vi "Enable Routing Channel.vi"(8 "error in (no error)":errorcluster, 11 "Channel Ref in":T1 format="%.0x") -> (0 "error out":errorcluster, 3 "Channel Ref out":T1 format="%.0x")   [LabVIEW 2017, in "Routing and Faulting Scripting.lvlib"]
uses:
  Routing and Faulting Scripting.lvlib
  <vilib>/NI Veristand/Custom Device API/Custom Device Item Ref.ctl
  <vilib>/NI Veristand/Custom Device API/Custom Device API.lvlib
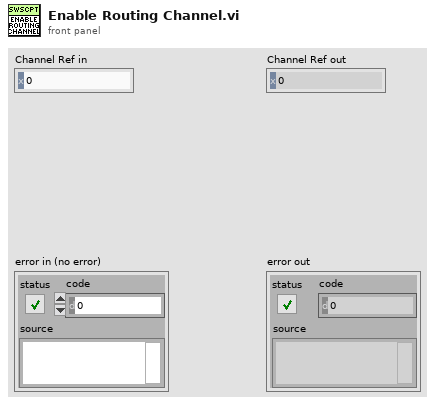
[diagram p1: front panel]
types:
  T1 = typedef "Custom Device API.lvlib/Custom Device Item Ref.ctl" = u64
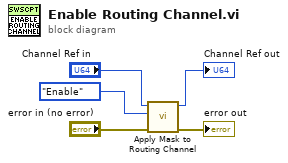
[diagram p0: block diagram]
diagram:
  n1 = call "Apply Mask to Routing Channel.vi"("error in (no error)"="error in (no error)", "Mask"=enum16{"Disable", "Enable"}."Enable", "Channel Ref in"="Channel Ref in") -> ("error out"=→"error out":errorcluster, "Channel Ref out"=→"Channel Ref out":T1)  [unwired: 7 in]
